vi "GetUIRef.vi"(8 "error in (no error)":errorcluster, 11 "View in":refnum<class "View.lvclass">) -> (0 "error out":errorcluster, 2 "VIRef":refnum<vi>, 3 "View out":refnum<class "View.lvclass">)   [LabVIEW 2020, in "UIHome.lvlib" / "View.lvclass"]
uses:
  View.lvclass
  View.lvclass/View.ctl
  UserInterface.vi
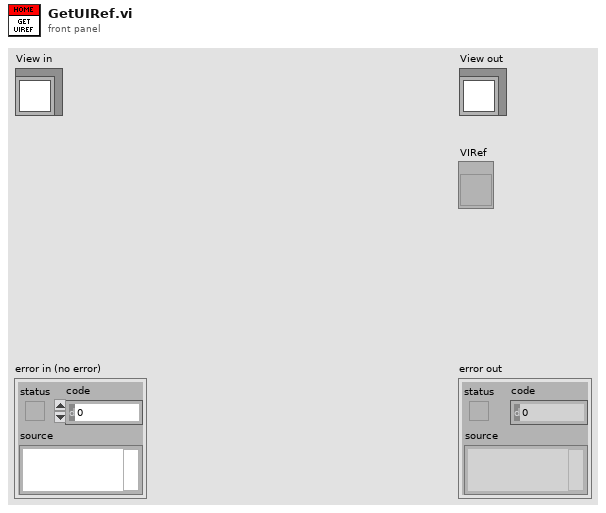
[diagram p1: front panel]
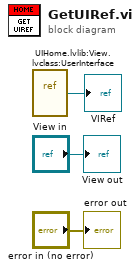
[diagram p0: block diagram]
diagram:
  n1 = vi-ref "UIHome.lvlib:View.lvclass:UserInterface.vi"() -> (→"VIRef":refnum<vi>)
  "error out" <- "error in (no error)"
  "View out" <- "View in"
